vi "Decimate DFD (Multistage).vi"(8 "error in (no error)":errorcluster, 10 "Decimation Factor":i32, 11 "Waveforms in":waveform(dbl)[](array[waveform])) -> (0 "error out":errorcluster, 3 "waveforms out":waveform(dbl)[](array[waveform]))   [LabVIEW 2019, in "DSP.lvclass"]
uses:
  DSP.lvclass
  <vilib>/Analysis/2dsp.llb/Decimate (single shot, DBL).vi
  <vilib>/Analysis/NI_AALPro.lvlib
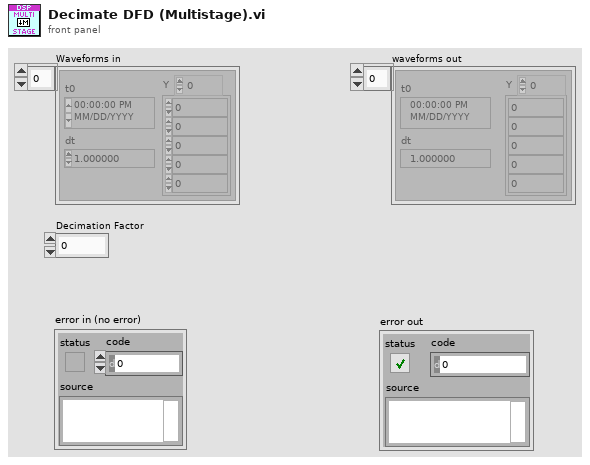
[diagram p1: front panel]
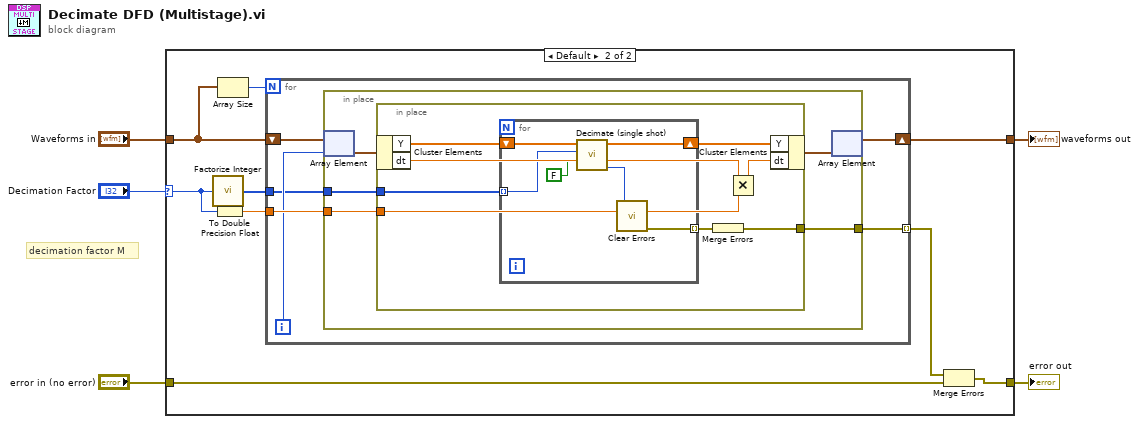
[diagram p0: block diagram]
diagram:
  # "decimation factor M"
  n1 = case shown="Default" "Decimation Factor" {
    selector: "Decimation Factor" -> [_ w9]
    tunnel: "Waveforms in" -> [w7 w10]
    tunnel: [w7 w16] -> w5
    tunnel: [w6 w15] -> w3
    tunnel: "error in (no error)" -> [w6 w14]
    frame 0, 1 {
    }
    frame Default {
      n2 = call "Factorize Integer.vi"("Integer in"=w9) -> ("Integer Factors"=w8:i32[])
      n3 = To Double Precision Float(number=w9) -> (double precision float=w11:dbl)
      n4 = Array Size(array=w10) -> (size(s)=w12:i32)
      n5 = for {
        N: w12 -> [_]
        tunnel: w11 -> [w22]
        tunnel: [w21] -> w13 mode=indexing
        shift-right: [w18] -> w16
        shift-left: w10 -> [w20]
        tunnel: w8 -> [w17]
        i -> [w19]
        n6 = in-place {
          in-place-border: w22 -> [w27]
          in-place-border: [w26] -> w21
          in-place-border: w17 -> [w25]
          n7 = in-place-array #1(w20, w19) -> (w24:waveform(dbl))
          n8 = in-place {
            in-place-border: w27 -> [w34]
            in-place-border: [w35] -> w26
            in-place-border: w25 -> [w28]
            n9 = in-place-cluster #2(w24) -> ("Y"=w32:dbl[], "dt"=w29:dbl)
            n10 = for {
              shift-right: [w40] -> w30
              shift-left: w32 -> [w41]
              tunnel: w28 -> [w39] mode=indexing
              tunnel: [w36] -> w33 mode=indexing
              n11 = call-poly <vilib>:"Decimate (single shot).vi"("averaging"=FALSE, "decimating factor"=w39, "X"=w41) -> ("error"=w37:i32, "Decimated Array"=w40:dbl[])  [unwired: 7 in]
              n12 = call <vilib>:"Clear Errors.vi"("specific error code to clear (0: all)"=w37) -> ("error out"=w36:errorcluster)  [unwired: 5 in, 1 out]
            }
            n13 = Merge Errors(w33) -> (w35:errorcluster)
            n14 = Multiply(x=w29, y=w34) -> (x*y=w31:dbl)
            n15 = in-place-cluster #2("Y"=w30, "dt"=w31) -> (w23:waveform(dbl))
          }
          n16 = in-place-array #1(w23) -> (w18:waveform(dbl)[])  [unwired: 1 out]
        }
      }
      n17 = Merge Errors(w13, w14) -> (w15:errorcluster)
    }
  }
  "waveforms out" <- w5
  "error out" <- w3
